vi "ST_parse_results_data.vi"(7 "data_start_index":i32, 8 "error_in":errorcluster, 11 "results_from_PLC":u8[](array[numeric])) -> (0 "error_out":errorcluster, 3 "results_from_PLC":T1)   [LabVIEW 2020]
uses:
  ST_results_info.ctl
  results_byte_offset/res_BATCH_offset.vi
  _misc/byte_array_parser/to_string.vi
  results_byte_offset/res_STRING_offset.vi
  results_byte_offset/res_REAL_offset.vi
  _misc/byte_array_parser/to_SGL.vi
  results_byte_offset/res_INT_offset.vi
  _misc/byte_array_parser/to_I16.vi
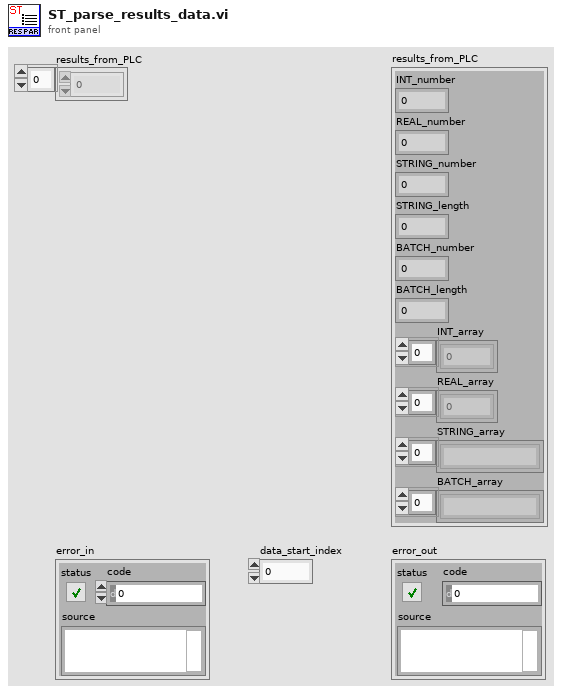
[diagram p1: front panel]
types:
  T1 = typedef "ST_results_info.ctl" = cluster{"INT_number":i32, "REAL_number":i32, "STRING_number":i32, "STRING_length":i32, "BATCH_number":i32, "BATCH_length":i32, "INT_array":i16[], "REAL_array":sgl[], "STRING_array":string[], "BATCH_array":string[]}
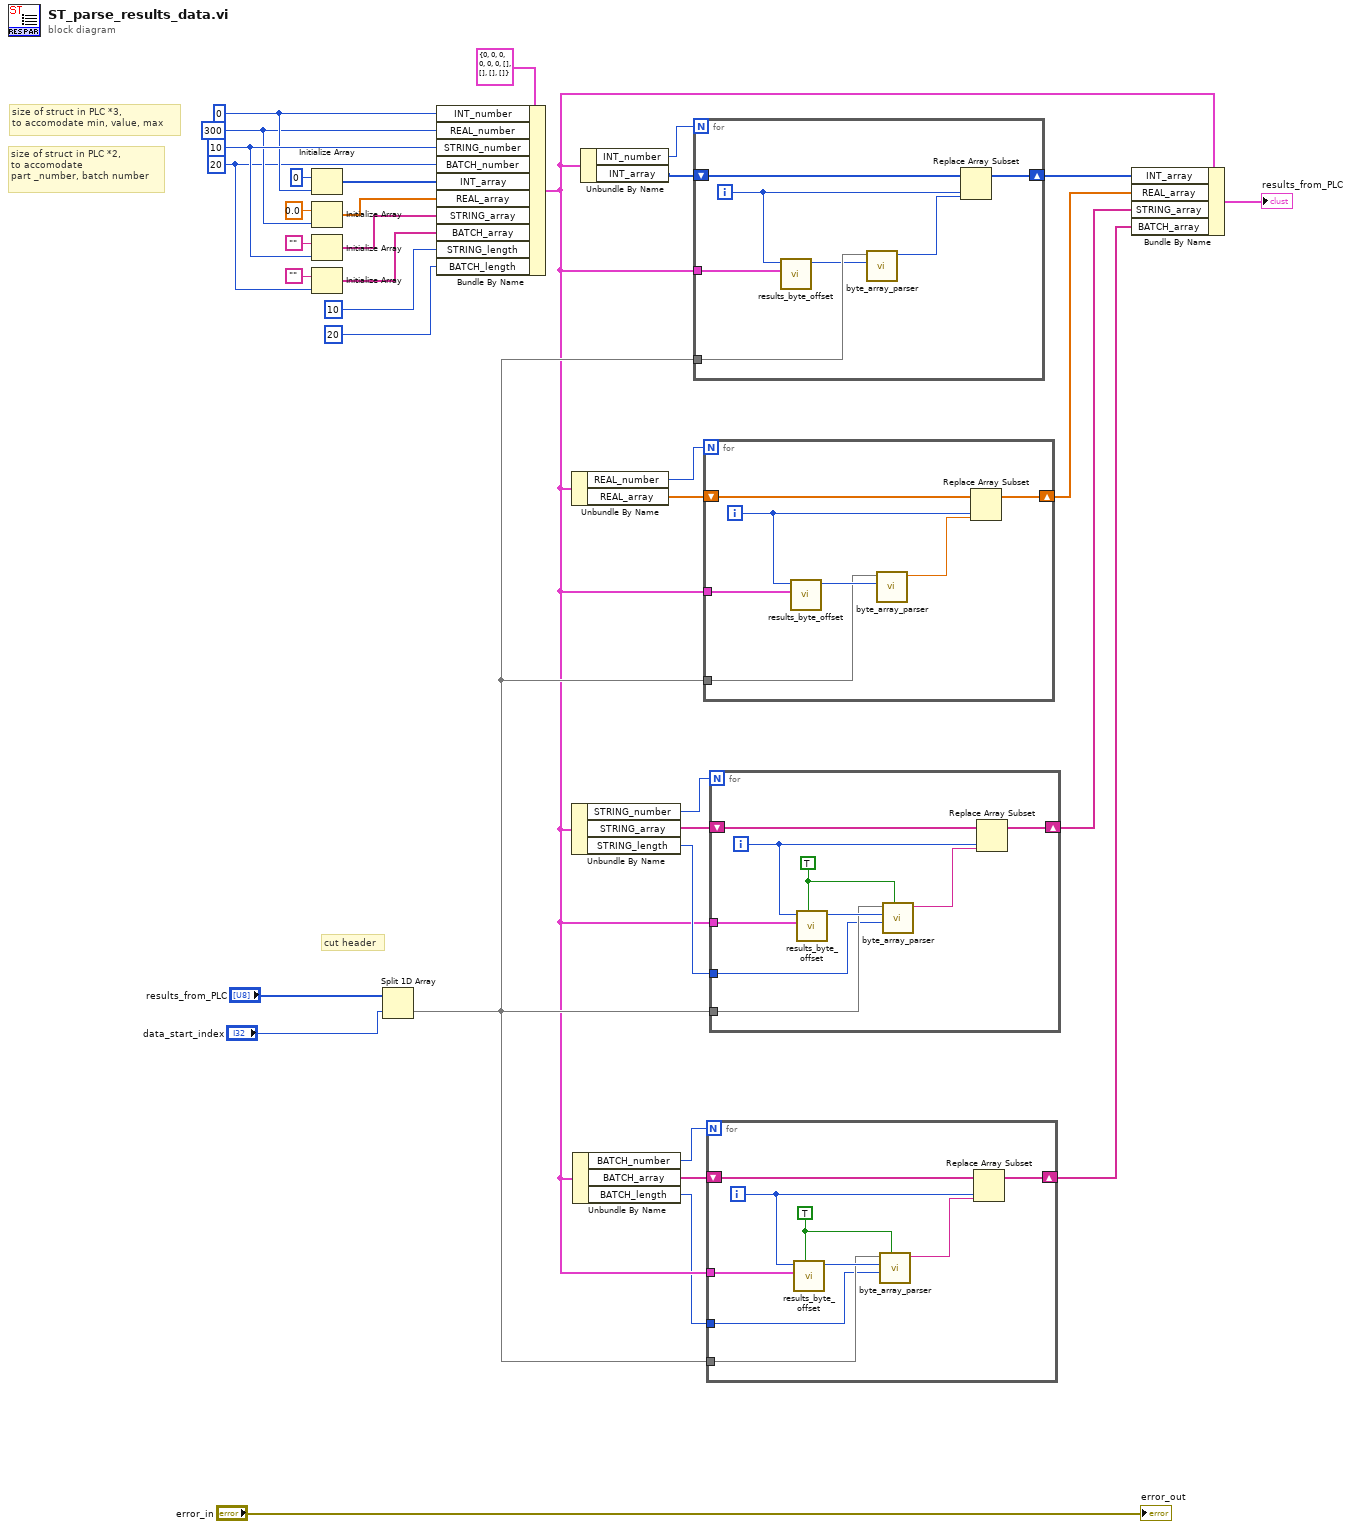
[diagram p0: block diagram]
diagram:
  w7 = 20 ("STRING_number")
  w30 = 10 ("STRING_number")
  w25 = 300 ("REAL_number")
  w26 = 0 ("INT_number")
  # "size of struct in PLC *2,\nto accomodate\npart _number, batch number"
  # "size of struct in PLC *3,\nto accomodate min, value, max"
  # "cut header"
  n1 = Initialize Array(i16 0 ("element"), w26) -> (w27:i16[])
  n2 = Initialize Array(sgl 0.0 ("element"), w25) -> (w28:sgl[])
  n3 = Initialize Array("", w30) -> (w29:string[])
  n4 = Initialize Array("", w7) -> (w8:string[])
  n5 = Split 1D Array(array="results_from_PLC", index="data_start_index") -> (second subarray=w6:u8[])  [unwired: 1 out]
  n6 = Bundle By Name(cluster=T1 {"INT_number"=0, "REAL_number"=0, "STRING_number"=0, "STRING_length"=0, "BATCH_number"=0, "BATCH_length"=0, "INT_array"=[], "REAL_array"=[], "STRING_array"=[], "BATCH_array"=[]} ("ST_reference_info"), "INT_number"=w26, "REAL_number"=w25, "STRING_number"=w30, "BATCH_number"=w7, "INT_array"=w27, "REAL_array"=w28, "STRING_array"=w29, "BATCH_array"=w8, "STRING_length"=10 ("y"), "BATCH_length"=20 ("y")) -> (w3:T1)
  n7 = Unbundle By Name(w3) -> ("REAL_number"=w22:i32, "REAL_array"=w21:sgl[])
  n8 = Unbundle By Name(w3) -> ("STRING_number"=w18:i32, "STRING_array"=w19:string[], "STRING_length"=w17:i32)
  n9 = Unbundle By Name(w3) -> ("BATCH_number"=w2:i32, "BATCH_array"=w4:string[], "BATCH_length"=w1:i32)
  n10 = Unbundle By Name(w3) -> ("INT_number"=w24:i32, "INT_array"=w23:i16[])
  n11 = for {
    N: w24 -> [_]
    shift-right: [w41] -> w20
    shift-left: w23 -> [w42]
    tunnel: w6 -> [w40]
    tunnel: w3 -> [w39]
    i -> [w36]
    n12 = call-poly "results_byte_offset.vi"("ST_results_info"=w39, "INT_position"=w36) -> ("results_byte_array_offset"=w38:i32)  [unwired: 9 in]
    n13 = call-poly "byte_array_parser.vi"("variable_start_index"=w38, "byte_array"=w40) -> ("I16"=w37:i16)  [unwired: 8 in, 1 out]
    n14 = Replace Array Subset(array=w42, new element=w37, index=w36) -> (w41:i16[])
  }
  n15 = for {
    N: w22 -> [_]
    shift-right: [w48] -> w14
    shift-left: w21 -> [w49]
    tunnel: w6 -> [w43]
    tunnel: w3 -> [w47]
    i -> [w44]
    n16 = call-poly "results_byte_offset.vi"("ST_results_info"=w47, "REAL_position"=w44) -> ("results_byte_array_offset"=w46:i32)  [unwired: 9 in]
    n17 = call-poly "byte_array_parser.vi"("variable_start_index"=w46, "byte_array"=w43) -> ("SGL"=w45:sgl)  [unwired: 8 in, 1 out]
    n18 = Replace Array Subset(array=w49, new element=w45, index=w44) -> (w48:sgl[])
  }
  n19 = for {
    N: w2 -> [_]
    shift-right: [w57] -> w5
    shift-left: w4 -> [w58]
    tunnel: w6 -> [w52]
    tunnel: w3 -> [w56]
    tunnel: w1 -> [w51]
    i -> [w53]
    w50 = TRUE ("Serialized by PLC? (F)")
    n20 = call-poly "results_byte_offset.vi"("Serialized by PLC? (F)"=w50, "ST_results_info"=w56, "BATCH_position"=w53) -> ("results_byte_array_offset"=w55:i32)  [unwired: 8 in]
    n21 = call-poly "byte_array_parser.vi"("Serialized by PLC? (F)"=w50, "string_length"=w51, "variable_start_index"=w55, "byte_array"=w52) -> ("string"=w54:string)  [unwired: 6 in, 1 out]
    n22 = Replace Array Subset(array=w58, new element=w54, index=w53) -> (w57:string[])
  }
  n23 = for {
    N: w18 -> [_]
    shift-right: [w66] -> w12
    shift-left: w19 -> [w67]
    tunnel: w6 -> [w61]
    tunnel: w3 -> [w65]
    tunnel: w17 -> [w60]
    i -> [w62]
    w59 = TRUE ("Serialized by PLC? (F)")
    n24 = call-poly "results_byte_offset.vi"("Serialized by PLC? (F)"=w59, "ST_results_info"=w65, "STRING_position"=w62) -> ("results_byte_array_offset"=w64:i32)  [unwired: 8 in]
    n25 = call-poly "byte_array_parser.vi"("Serialized by PLC? (F)"=w59, "string_length"=w60, "variable_start_index"=w64, "byte_array"=w61) -> ("string"=w63:string)  [unwired: 6 in, 1 out]
    n26 = Replace Array Subset(array=w67, new element=w63, index=w62) -> (w66:string[])
  }
  n27 = Bundle By Name(cluster=w3, "INT_array"=w20, "REAL_array"=w14, "STRING_array"=w12, "BATCH_array"=w5) -> (→"results_from_PLC":T1)
  "error_out" <- "error_in"
